vi "Color to HSL.vi"(2 "Color In":u32(colorbox)=16767232) -> (5 "H (degrees)":dbl, 6 "S (%)":dbl, 7 "L (%)":dbl, 8 "Hex":u32 format="%6x")   [LabVIEW 2021, in "Material SubVIs.lvlib"]
doc: "Convert color box input into HSL outputs\n\nBased on online converters testing methodology defined on wikepedia:\nhttps://www.rapidtables.com/convert/color/rgb-to-hsl.html\n\n<b>Code Developed By:</b> +\nDaniel Coons +\nTechnology Service Corporation +\nwww.tsc.com/atcs"
uses:
  Material SubVIs.lvlib
panel:
  out "R":u8
  out "G":u8
  out "B":u8
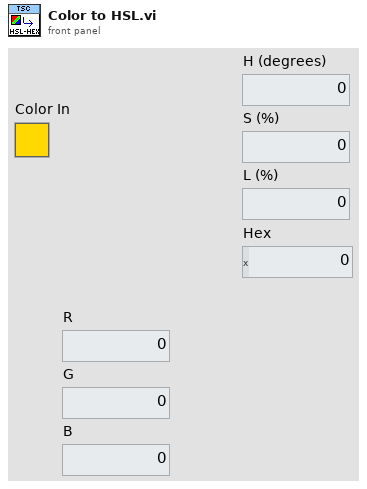
[diagram p1: front panel]
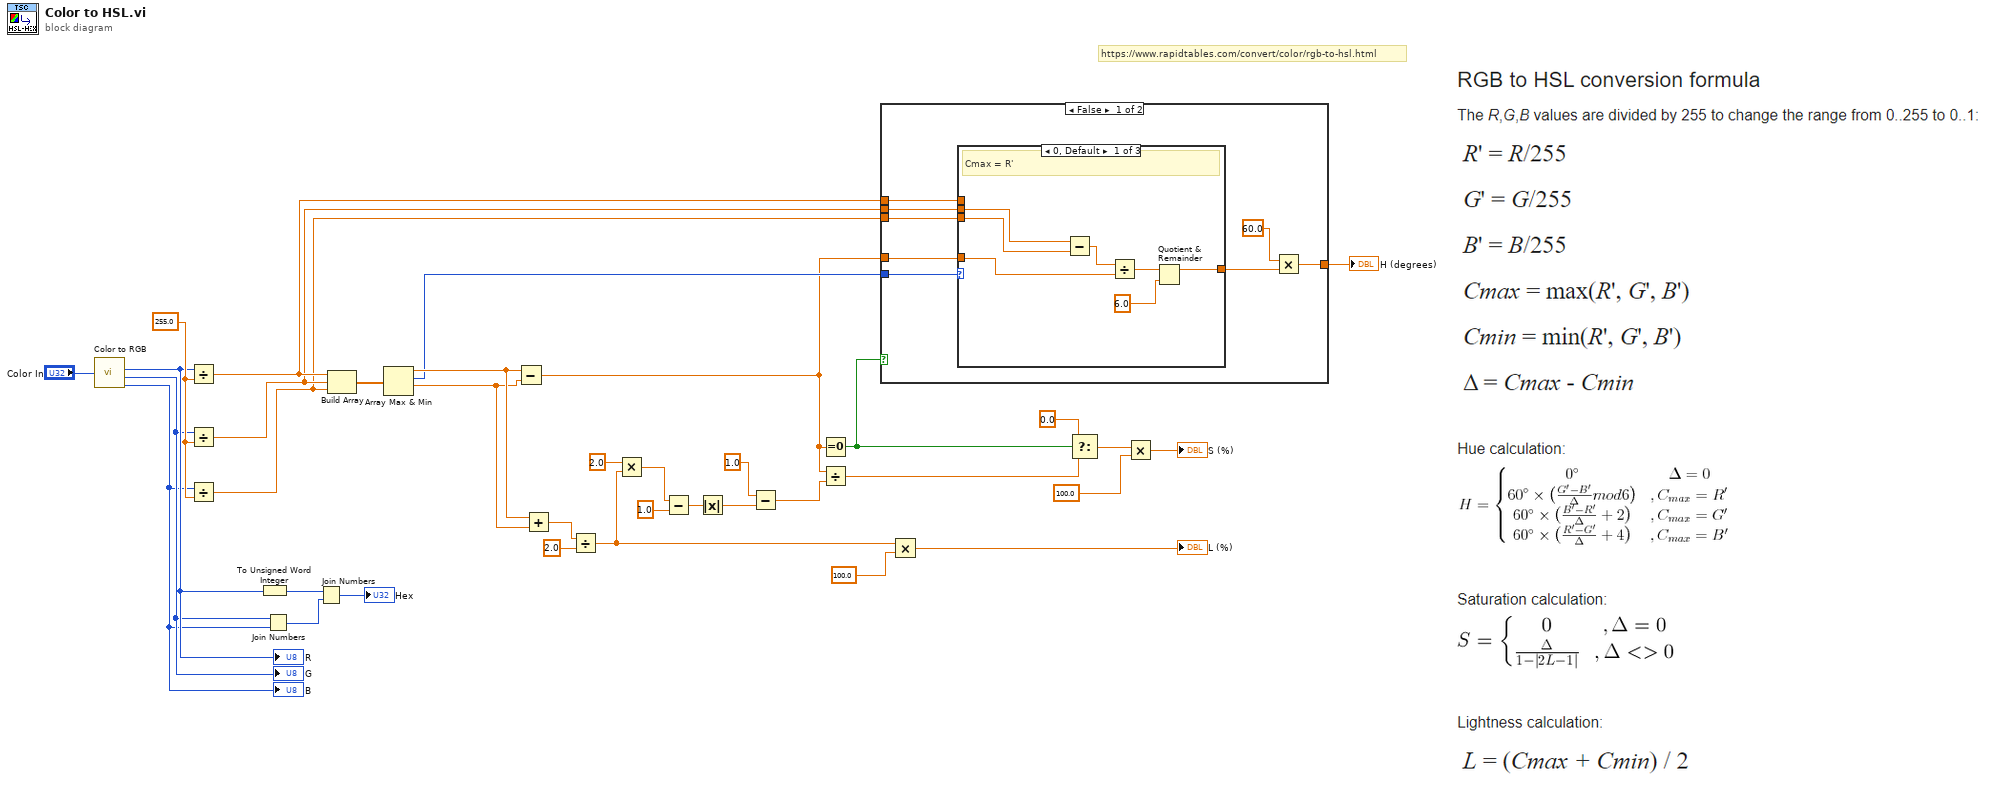
[diagram p0: block diagram]
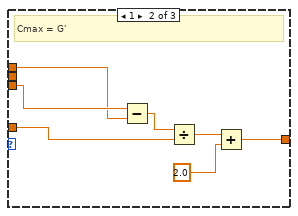
[diagram p2: hidden frame]
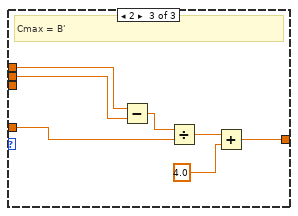
[diagram p3: hidden frame]
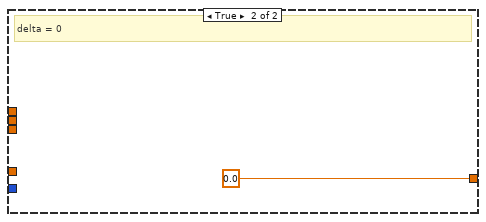
[diagram p4: hidden frame]
diagram:
  w34 = 255.0 ("y")
  # "https://www.rapidtables.com/convert/color/rgb-to-hsl.html"
  n1 = call <vilib>:"Color to RGB.vi"("Color"="Color In") -> ("R"=w3:u8, "G"=w2:u8, "B"=w1:u8)  [unwired: 1 out]
  "B" <- w1
  "G" <- w2
  "R" <- w3
  n2 = Divide(x=w3, y=w34) -> (x/y=w14:dbl)
  n3 = Divide(x=w2, y=w34) -> (x/y=w13:dbl)
  n4 = Divide(x=w1, y=w34) -> (x/y=w12:dbl)
  n5 = To Unsigned Word Integer(number=w3) -> (unsigned 16bit integer=w4:u16)
  n6 = Join Numbers(hi=w2, lo=w1) -> ((hi.lo)=w6:u16)
  n7 = Join Numbers(hi=w4, lo=w6) -> ((hi.lo)=→"Hex":u32)
  n8 = Build Array(w14, w13, w12) -> (w33:dbl[])
  n9 = Array Max & Min(array=w33) -> (max value=w32:dbl, max index (indices)=w15:i32, min value=w31:dbl)  [unwired: 1 out]
  n10 = Subtract(x=w32, y=w31) -> (x-y=w11:dbl)
  n11 = Add(x=w32, y=w31) -> (x+y=w30:dbl)
  n12 = Divide(x=w30, y=2.0) -> (x/y=w25:dbl)
  n13 = Multiply(x=2.0 ("y"), y=w25) -> (x*y=w23:dbl)
  n14 = Subtract(x=w23, y=1.0) -> (x-y=w21:dbl)
  n15 = Absolute Value(x=w21) -> (abs(x)=w20:dbl)
  n16 = Subtract(x=1.0, y=w20) -> (x-y=w19:dbl)
  n17 = Equal To 0?(x=w11) -> (x = 0?=w17:bool)
  n18 = Divide(x=w11, y=w19) -> (x/y=w18:dbl)
  n19 = case shown="False" w17 {
    tunnel: [w42 0.0 ("t")] -> w16
    tunnel: w15 -> [w43 _]
    tunnel: w14 -> [w39 _]
    tunnel: w13 -> [w38 _]
    tunnel: w12 -> [w37 _]
    tunnel: w11 -> [w36 _]
    frame False {
      n20 = case shown="0, Default" w43 {
        tunnel: [w44 w53 w60] -> w40
        tunnel: w39 -> [_ w51 w59]
        tunnel: w38 -> [w50 _ w58]
        tunnel: w37 -> [w49 w52 _]
        tunnel: w36 -> [w47 w56 w63]
        frame 0, Default {
          # "Cmax = R'"
          n21 = Subtract(x=w50, y=w49) -> (x-y=w48:dbl)
          n22 = Divide(x=w48, y=w47) -> (x/y=w46:dbl)
          n23 = Quotient & Remainder(x=w46, y=6.0) -> (x-y*floor(x/y)=w44:dbl)  [unwired: 1 out]
        }
        frame 1 {
          # "Cmax = G'"
          n24 = Subtract(x=w52, y=w51) -> (x-y=w57:dbl)
          n25 = Divide(x=w57, y=w56) -> (x/y=w55:dbl)
          n26 = Add(x=w55, y=2.0) -> (x+y=w53:dbl)
        }
        frame 2 {
          # "Cmax = B'"
          n27 = Subtract(x=w59, y=w58) -> (x-y=w64:dbl)
          n28 = Divide(x=w64, y=w63) -> (x/y=w62:dbl)
          n29 = Add(x=w62, y=4.0) -> (x+y=w60:dbl)
        }
      }
      n30 = Multiply(x=60.0, y=w40) -> (x*y=w42:dbl)
    }
    frame True {
      # "delta = 0"
    }
  }
  "H (degrees)" <- w16
  n31 = Multiply(x=w25, y=100.0) -> (x*y=→"L (%)":dbl)
  n32 = Select(t=0.0, s=w17, f=w18) -> (s? t:f=w28:dbl)
  n33 = Multiply(x=w28, y=100.0) -> (x*y=→"S (%)":dbl)
